vi "ULx Write (Digital 1D U16 NChan 1Samp).vi"(0 "task in":refnum<k24>, 1 "auto start":bool=TRUE, 7 "data":u16[](array[numeric]), 9 "timeout":dbl=10.0 format="%_4g", 11 "error in":errorcluster) -> (4 "task out":refnum<k24>, 10 "number of samples written per channel":u32, 15 "error out":errorcluster)   [LabVIEW 2020]
doc: "Writes a single 16-bit unsigned integer sample to a task that contains one or more digital output channels. Use an instance that writes 16-bit unsigned integers for devices with up to 16 lines per port."
uses:
  C:/Users/William/Documents/LV 2020 builds/LeaktestDAQ/Source-v33/ULx_LV.dll
  ULx_LV.dll
panel:
  # "channel"
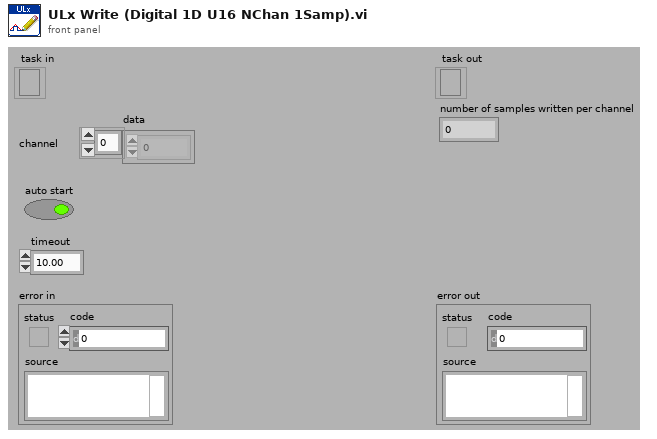
[diagram p1: front panel]
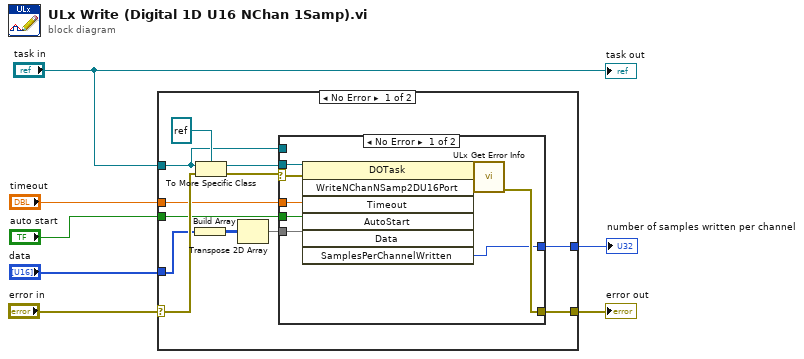
[diagram p0: block diagram]
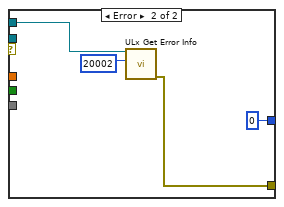
[diagram p2: hidden frame]
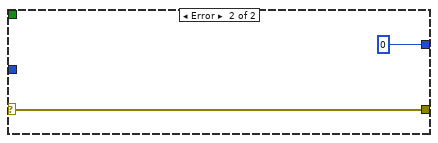
[diagram p3: hidden frame]
diagram:
  n1 = case shown="No Error" "error in" {
    selector: "error in" -> [w19 w35]
    tunnel: "task in" -> [w13 _]
    tunnel: "timeout" -> [w15 _]
    tunnel: [w14 w35] -> w5
    tunnel: "auto start" -> [w12 _]
    tunnel: [w11 0 ("SamplesPerChannelWritten")] -> w2
    tunnel: "data" -> [w10 _]
    frame No Error {
      n2 = Build Array(w10) -> (w9:u16[][])
      n3 = To More Specific Class(target class=refnum<k24> refnum, reference=w13, error in=w19) -> (specific class reference=w16:refnum<k24>, error out=w17:errorcluster)
      n4 = Transpose 2D Array(2D array=w9) -> (transposed array=w8:u16[][])
      n5 = case shown="No Error" w17 {
        selector: w17 -> [w28 _]
        tunnel: w16 -> [w29 _]
        tunnel: w15 -> [w22 _]
        tunnel: [w25 w32] -> w14
        tunnel: w13 -> [_ w31]
        tunnel: w12 -> [w21 _]
        tunnel: [w23 0 ("SamplesPerChannelWritten")] -> w11
        tunnel: w8 -> [w20 _]
        frame No Error {
          n6 = invoke class="DOTask" method="WriteNChanNSamp2DU16Port"(reference=w29, error in=w28, "Timeout"=w22, "AutoStart"=w21, "Data"=w20) -> (reference out=w26:refnum<k24>, error out=w27:errorcluster, "WriteNChanNSamp2DU16Port"=w24:i32, "SamplesPerChannelWritten"=w23:u32)  [unwired: 2 in, 3 out]
          n7 = call "ULx Get Error Info.vi"("error in"=w27, "ErrorCode"=w24, "task in"=w26) -> ("error out"=w25:errorcluster)  [unwired: 8 in]
        }
        frame Error {
          n8 = call "ULx Get Error Info.vi"("ErrorCode"=20002, "task in"=w31) -> ("error out"=w32:errorcluster)  [unwired: 9 in]
        }
      }
    }
    frame Error {
    }
  }
  "error out" <- w5
  "number of samples written per channel" <- w2
  "task out" <- "task in"
